vi "Extract Variable length miniscan pixels.vi"(8 "error in (no error)":errorcluster, 10 "ROI Coordinates (broken down to miniscans) out":T1, 11 "ROI Attributes (broken down to miniscans)":T2[](array[typedef]) {"Apparent Frame Size" format="%#_6f"; "Original FOV (um)" format="%#_6f"; "Pixels per miniscan" format="%#_6f"; "Dwell Time per pixel" format="%#_6f"; "Resolution" format="%#_6f"; "ROI group ID" format="%#_6f"; "Laser Power (%)" format="%#_6f"; "Zoom" format="%#_6f"; "Frame Size" format="%#_6f"; "Number of lines" format="%#_6f"; "Composite ID" format="%#_6f"; "Angle (deg)" format="%#_6f"; "ROI Time (ns)" format="%#_6f"; "ROI ID" format="%#_6f"; "Pixels in ROI" format="%#_6f"; "ROI index" format="%#_6f"; "Z stop" format="%#_6f"; "Y stop" format="%#_6f"; "X stop" format="%#_6f"; "Z start" format="%#_6f"; "X start" format="%#_6f"; "Y start" format="%#_6f"}) -> (0 "error out":errorcluster, 3 "Pixels per miniscan":u16[](array[numeric]))   [LabVIEW 2020]
uses:
  User Interface/Visualisation/Functional Imaging Viewer/Typedefs/ROI parameters data type.ctl
  Typedefs/ROI XY coordinates cluster.ctl
panel:
  out "Waveform Chart":u16[](graph)
  out "pixels array size":i32
  out "Coordinate array size":i32
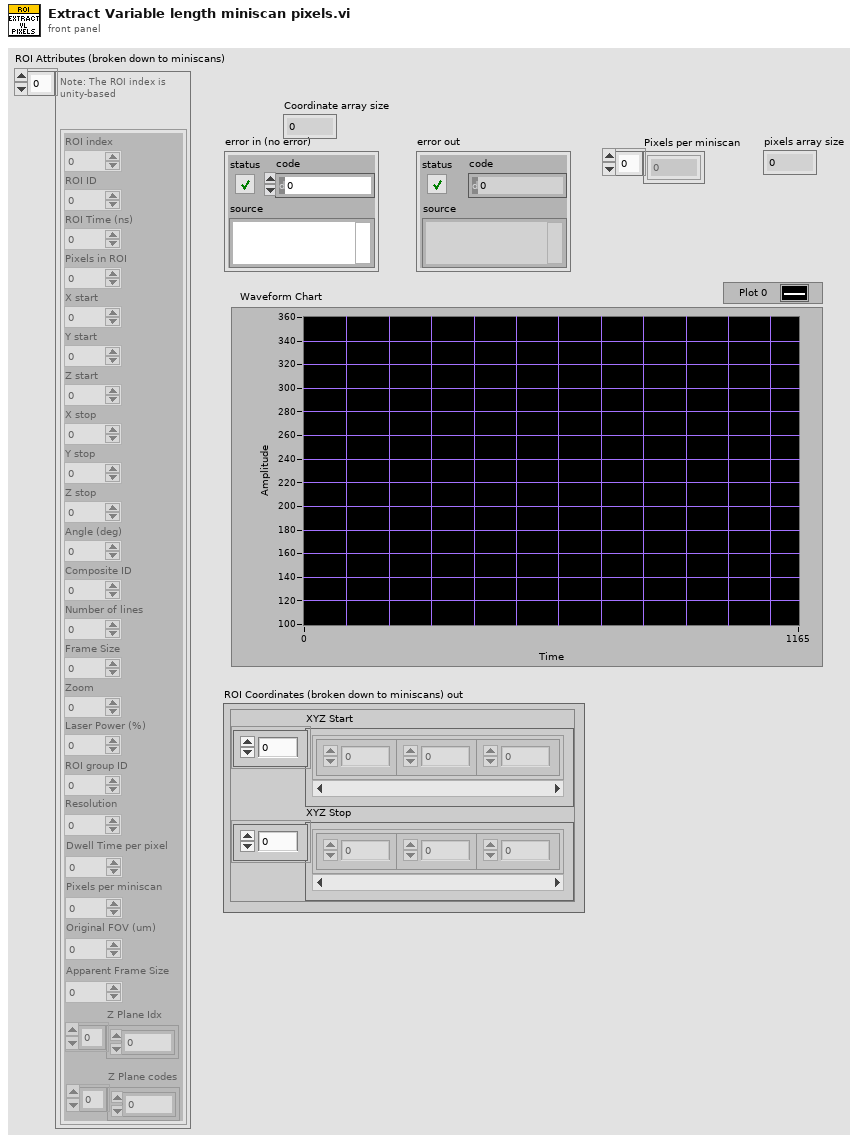
[diagram p1: front panel]
types:
  T1 = typedef "ROI XY coordinates cluster.ctl" = cluster{"XYZ Start":cluster{"X":sgl, "Y":sgl, "Z":sgl}[], "XYZ Stop":cluster{"X":sgl, "Y":sgl, "Z":sgl}[]}
  T2 = typedef "ROI parameters data type.ctl" = cluster{"ROI index":dbl, "ROI ID":dbl, "ROI Time (ns)":dbl, "Pixels in ROI":dbl, "X start":dbl, "Y start":dbl, "Z start":dbl, "X stop":dbl, "Y stop":dbl, "Z stop":dbl, "Angle (deg)":dbl, "Composite ID":dbl, "Number of lines":dbl, "Frame Size":dbl, "Zoom":dbl, "Laser Power (%)":dbl, "ROI group ID":dbl, "Resolution":dbl, "Dwell Time per pixel":dbl, "Pixels per miniscan":dbl, "Original FOV (um)":dbl, "Apparent Frame Size":dbl, "Z Plane Idx":i32[], "Z Plane codes":i32[]}
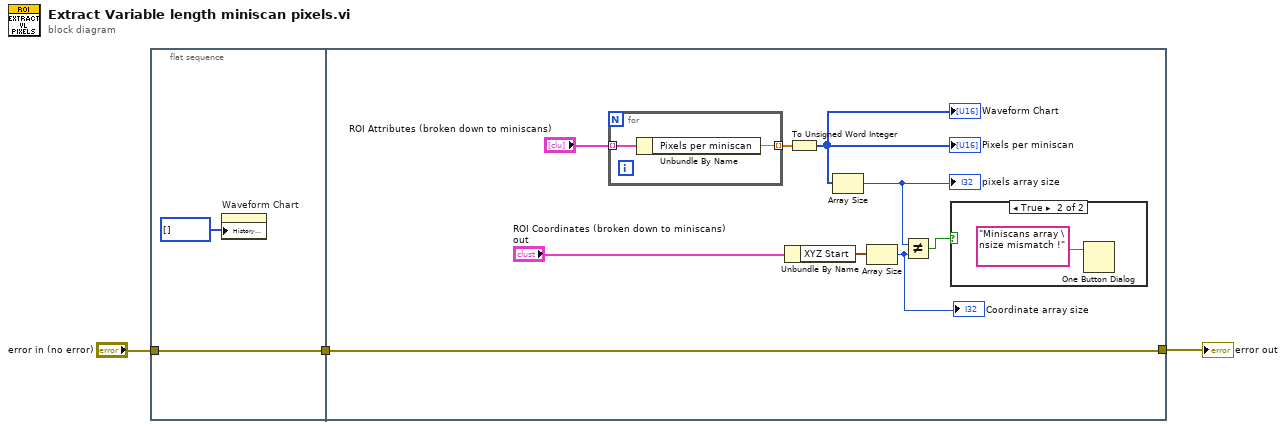
[diagram p0: block diagram]
diagram:
  n1 = flat-sequence {
    tunnel: "error in (no error)" -> [w5]
    tunnel: [w5] -> w1
    tunnel: [w6] -> w2
    tunnel: w1 -> [w6]
    frame #0 {
      n2 = property on="Waveform Chart" class="WFChart (strict)"("History Data"=u16[] []) -> ()  [unwired: 2 in, 2 out]
    }
    frame #1 {
      n3 = for {
        tunnel: "ROI Attributes (broken down to miniscans)" -> [w17] mode=indexing
        tunnel: [w16] -> w13 mode=indexing
        n4 = Unbundle By Name(w17) -> ("Pixels per miniscan"=w16:dbl)
      }
      n5 = Unbundle By Name("ROI Coordinates (broken down to miniscans) out") -> ("XYZ Start"=w11:cluster{"X":sgl, "Y":sgl, "Z":sgl}[])
      n6 = To Unsigned Word Integer(number=w13) -> (unsigned 16bit integer=w7:u16[])
      "Pixels per miniscan" <- w7
      "Waveform Chart" <- w7
      n7 = Array Size(array=w7) -> (size(s)=w10:i32)
      "pixels array size" <- w10
      n8 = Array Size(array=w11) -> (size(s)=w9:i32)
      "Coordinate array size" <- w9
      n9 = Not Equal?(x=w10, y=w9) -> (x != y?=w8:bool)
      n10 = case shown="True" w8 {
        frame False {
        }
        frame True {
          n11 = One Button Dialog(message="Miniscans array \nsize mismatch !") -> ()  [unwired: 1 in, 1 out]
        }
      }
    }
  }
  "error out" <- w2
